vi "deadband.vi"(1 "tolerance":dbl, 2 "input":dbl) -> (6 "output":dbl)   [LabVIEW 2011]
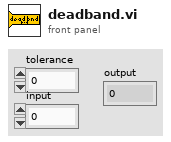
[diagram p1: front panel]
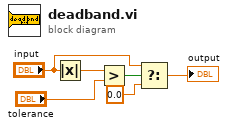
[diagram p0: block diagram]
diagram:
  n1 = Absolute Value(x="input") -> (abs(x)=w4:dbl)
  n2 = Greater?(x=w4, y="tolerance") -> (0:w6:bool)
  n3 = Select(t="input", s=w6, f=0.0) -> (s? t:f=→"output":dbl)
